vi "Enqueue FPGA.vi"(8 "error in (no error)":errorcluster, 10 "Data":variant, 11 "Command":string) -> (0 "error out":errorcluster, 3 "Queue Out":T1)   [LabVIEW 2023, in "FPGA.lvlib"]
uses:
  FPGA.lvlib
  Internal Communication/Controls/Queue.ctl
  Internal Communication/Internal Communication.lvlib
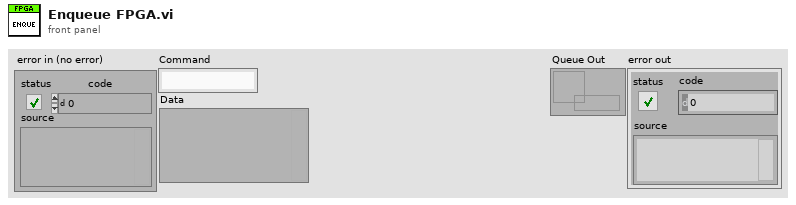
[diagram p1: front panel]
types:
  T1 = typedef "Queue.ctl" = refnum<queue>
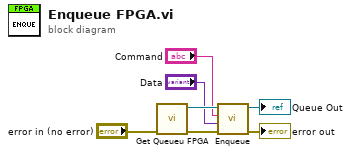
[diagram p0: block diagram]
diagram:
  n1 = call "Get Queueu FPGA.vi"("error in (no error)"="error in (no error)") -> ("error out"=w7:errorcluster, "Error Queue"=w6:refnum<queue>)  [unwired: 9 in]
  n2 = call "Enqueue.vi"("error in (no error)"=w7, "Data"="Data", "Command"="Command", "Queue In"=w6) -> ("error out"=→"error out":errorcluster, "Queue Out"=→"Queue Out":T1)  [unwired: 6 in]
